vi "PH_Numbers.round fractional digits.vi"(0 "Input":dbl format="%#_10g", 1 "Position (1)":i16=1) -> (2 "round Output":dbl format="%#_10g")   [LabVIEW 2014, in "PH_Common.lvlib"]
doc: "This VI rounds to the position after decimal point."
uses:
  PH_Common.lvlib
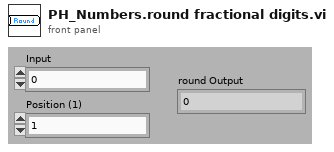
[diagram p1: front panel]
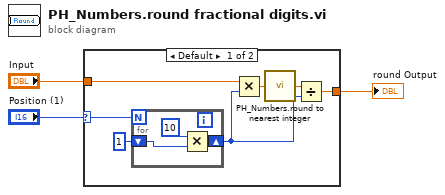
[diagram p0: block diagram]
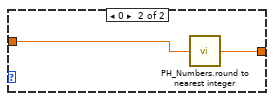
[diagram p2: hidden frame]
diagram:
  n1 = case shown="Default" "Position (1)" {
    selector: "Position (1)" -> [w4 _]
    tunnel: "Input" -> [w10 w15]
    tunnel: [w8 w14] -> w2
    frame Default {
      n2 = for {
        N: w4 -> [_]
        shift-right: [w13] -> w9
        shift-left: 1 -> [w11]
        n3 = Multiply(x=10, y=w11) -> (x*y=w13:i32)
      }
      n4 = Multiply(x=w10, y=w9) -> (x*y=w7:dbl)
      n5 = call "PH_Numbers.round to nearest integer.vi"("number"=w7) -> ("nearest integer value"=w6:dbl)
      n6 = Divide(x=w6, y=w9) -> (x/y=w8:dbl)
    }
    frame 0 {
      n7 = call "PH_Numbers.round to nearest integer.vi"("number"=w15) -> ("nearest integer value"=w14:dbl)
    }
  }
  "round Output" <- w2
